vi "FipsAdjacent.vi"() -> (11 "Fips":i32[](array[numeric]))   [LabVIEW 2017] (continued)
TN\"\t47041\n\"Warren County, TN\"\t47177\t\"Grundy County, TN\"\t47061\n\"Warren County, TN\"\t47177\t\"Sequatchie County, TN\"\t47153\n\"Warren County, TN\"\t47177\t\"Van Buren County, TN\"\t47175\n\"Warren County, TN\"\t47177\t\"Warren County, TN\"\t47177\n\"Warren County, TN\"\t47177\t\"White County, TN\"\t47185\n\"Washington County, TN\"\t47179\t\"Carter County, TN\"\t47019\n\"Washington County, TN\"\t47179\t\"Greene County, TN\"\t47059\n\"Washington County, TN\"\t47179\t\"Hawkins County, TN\"\t47073\n\"Washington County, TN\"\t47179\t\"Sullivan County, TN\"\t47163\n\"Washington County, TN\"\t47179\t\"Unicoi County, TN\"\t47171\n\"Washington County, TN\"\t47179\t\"Washington County, TN\"\t47179\n\"Wayne County, TN\"\t47181\t\"Lauderdale County, AL\"\t01077\n\"Wayne County, TN\"\t47181\t\"Decatur County, TN\"\t47039\n\"Wayne County, TN\"\t47181\t\"Hardin County, TN\"\t47071\n\"Wayne County, TN\"\t47181\t\"Lawrence County, TN\"\t47099\n\"Wayne County, TN\"\t47181\t\"Lewis County, TN\"\t47101\n\"Wayne County, TN\"\t47181\t\"Perry County, TN\"\t47135\n\"Wayne County, TN\"\t47181\t\"Wayne County, TN\"\t47181\n\"Weakley County, TN\"\t47183\t\"Graves County, KY\"\t21083\n\"Weakley County, TN\"\t47183\t\"Hickman County, KY\"\t21105\n\"Weakley County, TN\"\t47183\t\"Carroll County, TN\"\t47017\n\"Weakley County, TN\"\t47183\t\"Gibson County, TN\"\t47053\n\"Weakley County, TN\"\t47183\t\"Henry County, TN\"\t47079\n\"Weakley County, TN\"\t47183\t\"Obion County, TN\"\t47131\n\"Weakley County, TN\"\t47183\t\"Weakley County, TN\"\t47183\n\"White County, TN\"\t47185\t\"Cumberland County, TN\"\t47035\n\"White County, TN\"\t47185\t\"DeKalb County, TN\"\t47041\n\"White County, TN\"\t47185\t\"Putnam County, TN\"\t47141\n\"White County, TN\"\t47185\t\"Van Buren County, TN\"\t47175\n\"White County, TN\"\t47185\t\"Warren County, TN\"\t47177\n\"White County, TN\"\t47185\t\"White County, TN\"\t47185\n\"Williamson County, TN\"\t47187\t\"Cheatham County, TN\"\t47021\n\"Williamson County, TN\"\t47187\t\"Davidson County, TN\"\t47037\n\"Williamson County, TN\"\t47187\t\"Dickson County, TN\"\t47043\n\"Williamson County, TN\"\t47187\t\"Hickman County, TN\"\t47081\n\"Williamson County, TN\"\t47187\t\"Marshall County, TN\"\t47117\n\"Williamson County, TN\"\t47187\t\"Maury County, TN\"\t47119\n\"Williamson County, TN\"\t47187\t\"Rutherford County, TN\"\t47149\n\"Williamson County, TN\"\t47187\t\"Williamson County, TN\"\t47187\n\"Wilson County, TN\"\t47189\t\"Cannon County, TN\"\t47015\n\"Wilson County, TN\"\t47189\t\"Davidson County, TN\"\t47037\n\"Wilson County, TN\"\t47189\t\"DeKalb County, TN\"\t47041\n\"Wilson County, TN\"\t47189\t\"Rutherford County, TN\"\t47149\n\"Wilson County, TN\"\t47189\t\"Smith County, TN\"\t47159\n\"Wilson County, TN\"\t47189\t\"Sumner County, TN\"\t47165\n\"Wilson County, TN\"\t47189\t\"Trousdale County, TN\"\t47169\n\"Wilson County, TN\"\t47189\t\"Wilson County, TN\"\t47189\n\"Anderson County, TX\"\t48001\t\"Anderson County, TX\"\t48001\n\"Anderson County, TX\"\t48001\t\"Cherokee County, TX\"\t48073\n\"Anderson County, TX\"\t48001\t\"Freestone County, TX\"\t48161\n\"Anderson County, TX\"\t48001\t\"Henderson County, TX\"\t48213\n\"Anderson County, TX\"\t48001\t\"Houston County, TX\"\t48225\n\"Anderson County, TX\"\t48001\t\"Leon County, TX\"\t48289\n\"Andrews County, TX\"\t48003\t\"Lea County, NM\"\t35025\n\"Andrews County, TX\"\t48003\t\"Andrews County, TX\"\t48003\n\"Andrews County, TX\"\t48003\t\"Ector County, TX\"\t48135\n\"Andrews County, TX\"\t48003\t\"Gaines County, TX\"\t48165\n\"Andrews County, TX\"\t48003\t\"Martin County, TX\"\t48317\n\"Andrews County, TX\"\t48003\t\"Midland County, TX\"\t48329\n\"Andrews County, TX\"\t48003\t\"Winkler County, TX\"\t48495\n\"Angelina County, TX\"\t48005\t\"Angelina County, TX\"\t48005\n\"Angelina County, TX\"\t48005\t\"Cherokee County, TX\"\t48073\n\"Angelina County, TX\"\t48005\t\"Houston County, TX\"\t48225\n\"Angelina County, TX\"\t48005\t\"Jasper County, TX\"\t48241\n\"Angelina County, TX\"\t48005\t\"Nacogdoches County, TX\"\t48347\n\"Angelina County, TX\"\t48005\t\"Polk County, TX\"\t48373\n\"Angelina County, TX\"\t48005\t\"San Augustine County, TX\"\t48405\n\"Angelina County, TX\"\t48005\t\"Trinity County, TX\"\t48455\n\"Angelina County, TX\"\t48005\t\"Tyler County, TX\"\t48457\n\"Aransas County, TX\"\t48007\t\"Aransas County, TX\"\t48007\n\"Aransas County, TX\"\t48007\t\"Calhoun County, TX\"\t48057\n\"Aransas County, TX\"\t48007\t\"Nueces County, TX\"\t48355\n\"Aransas County, TX\"\t48007\t\"Refugio County, TX\"\t48391\n\"Aransas County, TX\"\t48007\t\"San Patricio County, TX\"\t48409\n\"Archer County, TX\"\t48009\t\"Archer County, TX\"\t48009\n\"Archer County, TX\"\t48009\t\"Baylor County, TX\"\t48023\n\"Archer County, TX\"\t48009\t\"Clay County, TX\"\t48077\n\"Archer County, TX\"\t48009\t\"Jack County, TX\"\t48237\n\"Archer County, TX\"\t48009\t\"Throckmorton County, TX\"\t48447\n\"Archer County, TX\"\t48009\t\"Wichita County, TX\"\t48485\n\"Archer County, TX\"\t48009\t\"Wilbarger County, TX\"\t48487\n\"Archer County, TX\"\t48009\t\"Young County, TX\"\t48503\n\"Armstrong County, TX\"\t48011\t\"Armstrong County, TX\"\t48011\n\"Armstrong County, TX\"\t48011\t\"Briscoe County, TX\"\t48045\n\"Armstrong County, TX\"\t48011\t\"Carson County, TX\"\t48065\n\"Armstrong County, TX\"\t48011\t\"Donley County, TX\"\t48129\n\"Armstrong County, TX\"\t48011\t\"Gray County, TX\"\t48179\n\"Armstrong County, TX\"\t48011\t\"Potter County, TX\"\t48375\n\"Armstrong County, TX\"\t48011\t\"Randall County, TX\"\t48381\n\"Armstrong County, TX\"\t48011\t\"Swisher County, TX\"\t48437\n\"Atascosa County, TX\"\t48013\t\"Atascosa County, TX\"\t48013\n\"Atascosa County, TX\"\t48013\t\"Bexar County, TX\"\t48029\n\"Atascosa County, TX\"\t48013\t\"Frio County, TX\"\t48163\n\"Atascosa County, TX\"\t48013\t\"Karnes County, TX\"\t48255\n\"Atascosa County, TX\"\t48013\t\"La Salle County, TX\"\t48283\n\"Atascosa County, TX\"\t48013\t\"Live Oak County, TX\"\t48297\n\"Atascosa County, TX\"\t48013\t\"McMullen County, TX\"\t48311\n\"Atascosa County, TX\"\t48013\t\"Medina County, TX\"\t48325\n\"Atascosa County, TX\"\t48013\t\"Wilson County, TX\"\t48493\n\"Austin County, TX\"\t48015\t\"Austin County, TX\"\t48015\n\"Austin County, TX\"\t48015\t\"Colorado County, TX\"\t48089\n\"Austin County, TX\"\t48015\t\"Fayette County, TX\"\t48149\n\"Austin County, TX\"\t48015\t\"Fort Bend County, TX\"\t48157\n\"Austin County, TX\"\t48015\t\"Waller County, TX\"\t48473\n\"Austin County, TX\"\t48015\t\"Washington County, TX\"\t48477\n\"Austin County, TX\"\t48015\t\"Wharton County, TX\"\t48481\n\"Bailey County, TX\"\t48017\t\"Curry County, NM\"\t35009\n\"Bailey County, TX\"\t48017\t\"Roosevelt County, NM\"\t35041\n\"Bailey County, TX\"\t48017\t\"Bailey County, TX\"\t48017\n\"Bailey County, TX\"\t48017\t\"Cochran County, TX\"\t48079\n\"Bailey County, TX\"\t48017\t\"Hockley County, TX\"\t48219\n\"Bailey County, TX\"\t48017\t\"Lamb County, TX\"\t48279\n\"Bailey County, TX\"\t48017\t\"Parmer County, TX\"\t48369\n\"Bandera County, TX\"\t48019\t\"Bandera County, TX\"\t48019\n\"Bandera County, TX\"\t48019\t\"Bexar County, TX\"\t48029\n\"Bandera County, TX\"\t48019\t\"Kendall County, TX\"\t48259\n\"Bandera County, TX\"\t48019\t\"Kerr County, TX\"\t48265\n\"Bandera County, TX\"\t48019\t\"Medina County, TX\"\t48325\n\"Bandera County, TX\"\t48019\t\"Real County, TX\"\t48385\n\"Bandera County, TX\"\t48019\t\"Uvalde County, TX\"\t48463\n\"Bastrop County, TX\"\t48021\t\"Bastrop County, TX\"\t48021\n\"Bastrop County, TX\"\t48021\t\"Caldwell County, TX\"\t48055\n\"Bastrop County, TX\"\t48021\t\"Fayette County, TX\"\t48149\n\"Bastrop County, TX\"\t48021\t\"Lee County, TX\"\t48287\n\"Bastrop County, TX\"\t48021\t\"Travis County, TX\"\t48453\n\"Bastrop County, TX\"\t48021\t\"Williamson County, TX\"\t48491\n\"Baylor County, TX\"\t48023\t\"Archer County, TX\"\t48009\n\"Baylor County, TX\"\t48023\t\"Baylor County, TX\"\t48023\n\"Baylor County, TX\"\t48023\t\"Foard County, TX\"\t48155\n\"Baylor County, TX\"\t48023\t\"Haskell County, TX\"\t48207\n\"Baylor County, TX\"\t48023\t\"Knox County, TX\"\t48275\n\"Baylor County, TX\"\t48023\t\"Throckmorton County, TX\"\t48447\n\"Baylor County, TX\"\t48023\t\"Wichita County, TX\"\t48485\n\"Baylor County, TX\"\t48023\t\"Wilbarger County, TX\"\t48487\n\"Baylor County, TX\"\t48023\t\"Young County, TX\"\t48503\n\"Bee County, TX\"\t48025\t\"Bee County, TX\"\t48025\n\"Bee County, TX\"\t48025\t\"Goliad County, TX\"\t48175\n\"Bee County, TX\"\t48025\t\"Karnes County, TX\"\t48255\n\"Bee County, TX\"\t48025\t\"Live Oak County, TX\"\t48297\n\"Bee County, TX\"\t48025\t\"Refugio County, TX\"\t48391\n\"Bee County, TX\"\t48025\t\"San Patricio County, TX\"\t48409\n\"Bell County, TX\"\t48027\t\"Bell County, TX\"\t48027\n\"Bell County, TX\"\t48027\t\"Burnet County, TX\"\t48053\n\"Bell County, TX\"\t48027\t\"Coryell County, TX\"\t48099\n\"Bell County, TX\"\t48027\t\"Falls County, TX\"\t48145\n\"Bell County, TX\"\t48027\t\"Lampasas County, TX\"\t48281\n\"Bell County, TX\"\t48027\t\"McLennan County, TX\"\t48309\n\"Bell County, TX\"\t48027\t\"Milam County, TX\"\t48331\n\"Bell County, TX\"\t48027\t\"Williamson County, TX\"\t48491\n\"Bexar County, TX\"\t48029\t\"Atascosa County, TX\"\t48013\n\"Bexar County, TX\"\t48029\t\"Bandera County, TX\"\t48019\n\"Bexar County, TX\"\t48029\t\"Bexar County, TX\"\t48029\n\"Bexar County, TX\"\t48029\t\"Comal County, TX\"\t48091\n\"Bexar County, TX\"\t48029\t\"Guadalupe County, TX\"\t48187\n\"Bexar County, TX\"\t48029\t\"Kendall County, TX\"\t48259\n\"Bexar County, TX\"\t48029\t\"Medina County, TX\"\t48325\n\"Bexar County, TX\"\t48029\t\"Wilson County, TX\"\t48493\n\"Blanco County, TX\"\t48031\t\"Blanco County, TX\"\t48031\n\"Blanco County, TX\"\t48031\t\"Burnet County, TX\"\t48053\n\"Blanco County, TX\"\t48031\t\"Comal County, TX\"\t48091\n\"Blanco County, TX\"\t48031\t\"Gillespie County, TX\"\t48171\n\"Blanco County, TX\"\t48031\t\"Hays County, TX\"\t48209\n\"Blanco County, TX\"\t48031\t\"Kendall County, TX\"\t48259\n\"Blanco County, TX\"\t48031\t\"Llano County, TX\"\t48299\n\"Blanco County, TX\"\t48031\t\"Travis County, TX\"\t48453\n\"Borden County, TX\"\t48033\t\"Borden County, TX\"\t48033\n\"Borden County, TX\"\t48033\t\"Dawson County, TX\"\t48115\n\"Borden County, TX\"\t48033\t\"Garza County, TX\"\t48169\n\"Borden County, TX\"\t48033\t\"Howard County, TX\"\t48227\n\"Borden County, TX\"\t48033\t\"Lynn County, TX\"\t48305\n\"Borden County, TX\"\t48033\t\"Martin County, TX\"\t48317\n\"Borden County, TX\"\t48033\t\"Mitchell County, TX\"\t48335\n\"Borden County, TX\"\t48033\t\"Scurry County, TX\"\t48415\n\"Bosque County, TX\"\t48035\t\"Bosque County, TX\"\t48035\n\"Bosque County, TX\"\t48035\t\"Coryell County, TX\"\t48099\n\"Bosque County, TX\"\t48035\t\"Erath County, TX\"\t48143\n\"Bosque County, TX\"\t48035\t\"Hamilton County, TX\"\t48193\n\"Bosque County, TX\"\t48035\t\"Hill County, TX\"\t48217\n\"Bosque County, TX\"\t48035\t\"Johnson County, TX\"\t48251\n\"Bosque County, TX\"\t48035\t\"McLennan County, TX\"\t48309\n\"Bosque County, TX\"\t48035\t\"Somervell County, TX\"\t48425\n\"Bowie County, TX\"\t48037\t\"Little River County, AR\"\t05081\n\"Bowie County, TX\"\t48037\t\"Miller County, AR\"\t05091\n\"Bowie County, TX\"\t48037\t\"McCurtain County, OK\"\t40089\n\"Bowie County, TX\"\t48037\t\"Bowie County, TX\"\t48037\n\"Bowie County, TX\"\t48037\t\"Cass County, TX\"\t48067\n\"Bowie County, TX\"\t48037\t\"Morris County, TX\"\t48343\n\"Bowie County, TX\"\t48037\t\"Red River County, TX\"\t48387\n\"Brazoria County, TX\"\t48039\t\"Brazoria County, TX\"\t48039\n\"Brazoria County, TX\"\t48039\t\"Fort Bend County, TX\"\t48157\n\"Brazoria County, TX\"\t48039\t\"Galveston County, TX\"\t48167\n\"Brazoria County, TX\"\t48039\t\"Harris County, TX\"\t48201\n\"Brazoria County, TX\"\t48039\t\"Matagorda County, TX\"\t48321\n\"Brazoria County, TX\"\t48039\t\"Wharton County, TX\"\t48481\n\"Brazos County, TX\"\t48041\t\"Brazos County, TX\"\t48041\n\"Brazos County, TX\"\t48041\t\"Burleson County, TX\"\t48051\n\"Brazos County, TX\"\t48041\t\"Grimes County, TX\"\t48185\n\"Brazos County, TX\"\t48041\t\"Leon County, TX\"\t48289\n\"Brazos County, TX\"\t48041\t\"Madison County, TX\"\t48313\n\"Brazos County, TX\"\t48041\t\"Robertson County, TX\"\t48395\n\"Brazos County, TX\"\t48041\t\"Washington County, TX\"\t48477\n\"Brewster County, TX\"\t48043\t\"Brewster County, TX\"\t48043\n\"Brewster County, TX\"\t48043\t\"Jeff Davis County, TX\"\t48243\n\"Brewster County, TX\"\t48043\t\"Pecos County, TX\"\t48371\n\"Brewster County, TX\"\t48043\t\"Presidio County, TX\"\t48377\n\"Brewster County, TX\"\t48043\t\"Terrell County, TX\"\t48443\n\"Briscoe County, TX\"\t48045\t\"Armstrong County, TX\"\t48011\n\"Briscoe County, TX\"\t48045\t\"Briscoe County, TX\"\t48045\n\"Briscoe County, TX\"\t48045\t\"Donley County, TX\"\t48129\n\"Briscoe County, TX\"\t48045\t\"Floyd County, TX\"\t48153\n\"Briscoe County, TX\"\t48045\t\"Hall County, TX\"\t48191\n\"Briscoe County, TX\"\t48045\t\"Motley County, TX\"\t48345\n\"Briscoe County, TX\"\t48045\t\"Swisher County, TX\"\t48437\n\"Brooks County, TX\"\t48047\t\"Brooks County, TX\"\t48047\n\"Brooks County, TX\"\t48047\t\"Duval County, TX\"\t48131\n\"Brooks County, TX\"\t48047\t\"Hidalgo County, TX\"\t48215\n\"Brooks County, TX\"\t48047\t\"Jim Hogg County, TX\"\t48247\n\"Brooks County, TX\"\t48047\t\"Jim Wells County, TX\"\t48249\n\"Brooks County, TX\"\t48047\t\"Kenedy County, TX\"\t48261\n\"Brooks County, TX\"\t48047\t\"Kleberg County, TX\"\t48273\n\"Brooks County, TX\"\t48047\t\"Starr County, TX\"\t48427\n\"Brown County, TX\"\t48049\t\"Brown County, TX\"\t48049\n\"Brown County, TX\"\t48049\t\"Callahan County, TX\"\t48059\n\"Brown County, TX\"\t48049\t\"Coleman County, TX\"\t48083\n\"Brown County, TX\"\t48049\t\"Comanche County, TX\"\t48093\n\"Brown County, TX\"\t48049\t\"Eastland County, TX\"\t48133\n\"Brown County, TX\"\t48049\t\"McCulloch County, TX\"\t48307\n\"Brown County, TX\"\t48049\t\"Mills County, TX\"\t48333\n\"Brown County, TX\"\t48049\t\"San Saba County, TX\"\t48411\n\"Burleson County, TX\"\t48051\t\"Brazos County, TX\"\t48041\n\"Burleson County, TX\"\t48051\t\"Burleson County, TX\"\t48051\n\"Burleson County, TX\"\t48051\t\"Lee County, TX\"\t48287\n\"Burleson County, TX\"\t48051\t\"Milam County, TX\"\t48331\n\"Burleson County, TX\"\t48051\t\"Robertson County, TX\"\t48395\n\"Burleson County, TX\"\t48051\t\"Washington County, TX\"\t48477\n\"Burnet County, TX\"\t48053\t\"Bell County, TX\"\t48027\n\"Burnet County, TX\"\t48053\t\"Blanco County, TX\"\t48031\n\"Burnet County, TX\"\t48053\t\"Burnet County, TX\"\t48053\n\"Burnet County, TX\"\t48053\t\"Lampasas County, TX\"\t48281\n\"Burnet County, TX\"\t48053\t\"Llano County, TX\"\t48299\n\"Burnet County, TX\"\t48053\t\"San Saba County, TX\"\t48411\n\"Burnet County, TX\"\t48053\t\"Travis County, TX\"\t48453\n\"Burnet County, TX\"\t48053\t\"Williamson County, TX\"\t48491\n\"Caldwell County, TX\"\t48055\t\"Bastrop County, TX\"\t48021\n\"Caldwell County, TX\"\t48055\t\"Caldwell County, TX\"\t48055\n\"Caldwell County, TX\"\t48055\t\"Fayette County, TX\"\t48149\n\"Caldwell County, TX\"\t48055\t\"Gonzales County, TX\"\t48177\n\"Caldwell County, TX\"\t48055\t\"Guadalupe County, TX\"\t48187\n\"Caldwell County, TX\"\t48055\t\"Hays County, TX\"\t48209\n\"Caldwell County, TX\"\t48055\t\"Travis County, TX\"\t48453\n\"Calhoun County, TX\"\t48057\t\"Aransas County, TX\"\t48007\n\"Calhoun County, TX\"\t48057\t\"Calhoun County, TX\"\t48057\n\"Calhoun County, TX\"\t48057\t\"Jackson County, TX\"\t48239\n\"Calhoun County, TX\"\t48057\t\"Matagorda County, TX\"\t48321\n\"Calhoun County, TX\"\t48057\t\"Refugio County, TX\"\t48391\n\"Calhoun County, TX\"\t48057\t\"Victoria County, TX\"\t48469\n\"Callahan County, TX\"\t48059\t\"Brown County, TX\"\t48049\n\"Callahan County, TX\"\t48059\t\"Callahan County, TX\"\t48059\n\"Callahan County, TX\"\t48059\t\"Coleman County, TX\"\t48083\n\"Callahan County, TX\"\t48059\t\"Eastland County, TX\"\t48133\n\"Callahan County, TX\"\t48059\t\"Jones County, TX\"\t48253\n\"Callahan County, TX\"\t48059\t\"Shackelford County, TX\"\t48417\n\"Callahan County, TX\"\t48059\t\"Taylor County, TX\"\t48441\n\"Cameron County, TX\"\t48061\t\"Cameron County, TX\"\t48061\n\"Cameron County, TX\"\t48061\t\"Hidalgo County, TX\"\t48215\n\"Cameron County, TX\"\t48061\t\"Willacy County, TX\"\t48489\n\"Camp County, TX\"\t48063\t\"Camp County, TX\"\t48063\n\"Camp County, TX\"\t48063\t\"Franklin County, TX\"\t48159\n\"Camp County, TX\"\t48063\t\"Morris County, TX\"\t48343\n\"Camp County, TX\"\t48063\t\"Titus County, TX\"\t48449\n\"Camp County, TX\"\t48063\t\"Upshur County, TX\"\t48459\n\"Camp County, TX\"\t48063\t\"Wood County, TX\"\t48499\n\"Carson County, TX\"\t48065\t\"Armstrong County, TX\"\t48011\n\"Carson County, TX\"\t48065\t\"Carson County, TX\"\t48065\n\"Carson County, TX\"\t48065\t\"Donley County, TX\"\t48129\n\"Carson County, TX\"\t48065\t\"Gray County, TX\"\t48179\n\"Carson County, TX\"\t48065\t\"Hutchinson County, TX\"\t48233\n\"Carson County, TX\"\t48065\t\"Moore County, TX\"\t48341\n\"Carson County, TX\"\t48065\t\"Potter County, TX\"\t48375\n\"Carson County, TX\"\t48065\t\"Randall County, TX\"\t48381\n\"Carson County, TX\"\t48065\t\"Roberts County, TX\"\t48393\n\"Cass County, TX\"\t48067\t\"Miller County, AR\"\t05091\n\"Cass County, TX\"\t48067\t\"Caddo Parish, LA\"\t22017\n\"Cass County, TX\"\t48067\t\"Bowie County, TX\"\t48037\n\"Cass County, TX\"\t48067\t\"Cass County, TX\"\t48067\n\"Cass County, TX\"\t48067\t\"Marion County, TX\"\t48315\n\"Cass County, TX\"\t48067\t\"Morris County, TX\"\t48343\n\"Castro County, TX\"\t48069\t\"Castro County, TX\"\t48069\n\"Castro County, TX\"\t48069\t\"Deaf Smith County, TX\"\t48117\n\"Castro County, TX\"\t48069\t\"Hale County, TX\"\t48189\n\"Castro County, TX\"\t48069\t\"Lamb County, TX\"\t48279\n\"Castro County, TX\"\t48069\t\"Parmer County, TX\"\t48369\n\"Castro County, TX\"\t48069\t\"Randall County, TX\"\t48381\n\"Castro County, TX\"\t48069\t\"Swisher County, TX\"\t48437\n\"Chambers County, TX\"\t48071\t\"Chambers County, TX\"\t48071\n\"Chambers County, TX\"\t48071\t\"Galveston County, TX\"\t48167\n\"Chambers County, TX\"\t48071\t\"Harris County, TX\"\t48201\n\"Chambers County, TX\"\t48071\t\"Jefferson County, TX\"\t48245\n\"Chambers County, TX\"\t48071\t\"Liberty County, TX\"\t48291\n\"Cherokee County, TX\"\t48073\t\"Anderson County, TX\"\t48001\n\"Cherokee County, TX\"\t48073\t\"Angelina County, TX\"\t48005\n\"Cherokee County, TX\"\t48073\t\"Cherokee County, TX\"\t48073\n\"Cherokee County, TX\"\t48073\t\"Henderson County, TX\"\t48213\n\"Cherokee County, TX\"\t48073\t\"Houston County, TX\"\t48225\n\"Cherokee County, TX\"\t48073\t\"Nacogdoches County, TX\"\t48347\n\"Cherokee County, TX\"\t48073\t\"Rusk County, TX\"\t48401\n\"Cherokee County, TX\"\t48073\t\"Smith County, TX\"\t48423\n\"Childress County, TX\"\t48075\t\"Harmon County, OK\"\t40057\n\"Childress County, TX\"\t48075\t\"Childress County, TX\"\t48075\n\"Childress County, TX\"\t48075\t\"Collingsworth County, TX\"\t48087\n\"Childress County, TX\"\t48075\t\"Cottle County, TX\"\t48101\n\"Childress County, TX\"\t48075\t\"Hall County, TX\"\t48191\n\"Childress County, TX\"\t48075\t\"Hardeman County, TX\"\t48197\n\"Clay County, TX\"\t48077\t\"Cotton County, OK\"\t40033\n\"Clay County, TX\"\t48077\t\"Jefferson County, OK\"\t40067\n\"Clay County, TX\"\t48077\t\"Archer County, TX\"\t48009\n\"Clay County, TX\"\t48077\t\"Clay County, TX\"\t48077\n\"Clay County, TX\"\t48077\t\"Jack County, TX\"\t48237\n\"Clay County, TX\"\t48077\t\"Montague County, TX\"\t48337\n\"Clay County, TX\"\t48077\t\"Wichita County, TX\"\t48485\n\"Cochran County, TX\"\t48079\t\"Lea County, NM\"\t35025\n\"Cochran County, TX\"\t48079\t\"Roosevelt County, NM\"\t35041\n\"Cochran County, TX\"\t48079\t\"Bailey County, TX\"\t48017\n\"Cochran County, TX\"\t48079\t\"Cochran County, TX\"\t48079\n\"Cochran County, TX\"\t48079\t\"Hockley County, TX\"\t48219\n\"Cochran County, TX\"\t48079\t\"Lamb County, TX\"\t48279\n\"Cochran County, TX\"\t48079\t\"Terry County, TX\"\t48445\n\"Cochran County, TX\"\t48079\t\"Yoakum County, TX\"\t48501\n\"Coke County, TX\"\t48081\t\"Coke County, TX\"\t48081\n\"Coke County, TX\"\t48081\t\"Mitchell County, TX\"\t48335\n\"Coke County, TX\"\t48081\t\"Nolan County, TX\"\t48353\n\"Coke County, TX\"\t48081\t\"Runnels County, TX\"\t48399\n\"Coke County, TX\"\t48081\t\"Sterling County, TX\"\t48431\n\"Coke County, TX\"\t48081\t\"Tom Green County, TX\"\t48451\n\"Coleman County, TX\"\t48083\t\"Brown County, TX\"\t48049\n\"Coleman County, TX\"\t48083\t\"Callahan County, TX\"\t48059\n\"Coleman County, TX\"\t48083\t\"Coleman County, TX\"\t48083\n\"Coleman County, TX\"\t48083\t\"Concho County, TX\"\t48095\n\"Coleman County, TX\"\t48083\t\"McCulloch County, TX\"\t48307\n\"Coleman County, TX\"\t48083\t\"Runnels County, TX\"\t48399\n\"Coleman County, TX\"\t48083\t\"Taylor County, TX\"\t48441\n\"Collin County, TX\"\t48085\t\"Collin County, TX\"\t48085\n\"Collin County, TX\"\t48085\t\"Dallas County, TX\"\t48113\n\"Collin County, TX\"\t48085\t\"Denton County, TX\"\t48121\n\"Collin County, TX\"\t48085\t\"Fannin County, TX\"\t48147\n\"Collin County, TX\"\t48085\t\"Grayson County, TX\"\t48181\n\"Collin County, TX\"\t48085\t\"Hunt County, TX\"\t48231\n\"Collin County, TX\"\t48085\t\"Rockwall County, TX\"\t48397\n\"Collingsworth County, TX\"\t48087\t\"Beckham County, OK\"\t40009\n\"Collingsworth County, TX\"\t48087\t\"Harmon County, OK\"\t40057\n\"Collingsworth County, TX\"\t48087\t\"Childress County, TX\"\t48075\n\"Collingsworth County, TX\"\t48087\t\"Collingsworth County, TX\"\t48087\n\"Collingsworth County, TX\"\t48087\t\"Donley County, TX\"\t48129\n\"Collingsworth County, TX\"\t48087\t\"Gray County, TX\"\t48179\n\"Collingsworth County, TX\"\t48087\t\"Hall County, TX\"\t48191\n\"Collingsworth County, TX\"\t48087\t\"Wheeler County, TX\"\t48483\n\"Colorado County, TX\"\t48089\t\"Austin County, TX\"\t48015\n\"Colorado County, TX\"\t48089\t\"Colorado County, TX\"\t48089\n\"Colorado County, TX\"\t48089\t\"Fayette County, TX\"\t48149\n\"Colorado County, TX\"\t48089\t\"Jackson County, TX\"\t48239\n\"Colorado County, TX\"\t48089\t\"Lavaca County, TX\"\t48285\n\"Colorado County, TX\"\t48089\t\"Wharton County, TX\"\t48481\n\"Comal County, TX\"\t48091\t\"Bexar County, TX\"\t48029\n\"Comal County, TX\"\t48091\t\"Blanco County, TX\"\t48031\n\"Comal County, TX\"\t48091\t\"Comal County, TX\"\t48091\n\"Comal County, TX\"\t48091\t\"Guadalupe County, TX\"\t48187\n\"Comal County, TX\"\t48091\t\"Hays County, TX\"\t48209\n\"Comal County, TX\"\t48091\t\"Kendall County, TX\"\t48259\n\"Comanche County, TX\"\t48093\t\"Brown County, TX\"\t48049\n\"Comanche County, TX\"\t48093\t\"Comanche County, TX\"\t48093\n\"Comanche County, TX\"\t48093\t\"Eastland County, TX\"\t48133\n\"Comanche County, TX\"\t48093\t\"Erath County, TX\"\t48143\n\"Comanche County, TX\"\t48093\t\"Hamilton County, TX\"\t48193\n\"Comanche County, TX\"\t48093\t\"Mills County, TX\"\t48333\n\"Concho County, TX\"\t48095\t\"Coleman County, TX\"\t48083\n\"Concho County, TX\"\t48095\t\"Concho County, TX\"\t48095\n\"Concho County, TX\"\t48095\t\"McCulloch County, TX\"\t48307\n\"Concho County, TX\"\t48095\t\"Menard County, TX\"\t48327\n\"Concho County, TX\"\t48095\t\"Runnels County, TX\"\t48399\n\"Concho County, TX\"\t48095\t\"Schleicher County, TX\"\t48413\n\"Concho County, TX\"\t48095\t\"Tom Green County, TX\"\t48451\n\"Cooke County, TX\"\t48097\t\"Love County, OK\"\t40085\n\"Cooke County, TX\"\t48097\t\"Cooke County, TX\"\t48097\n\"Cooke County, TX\"\t48097\t\"Denton County, TX\"\t48121\n\"Cooke County, TX\"\t48097\t\"Grayson County, TX\"\t48181\n\"Cooke County, TX\"\t48097\t\"Montague County, TX\"\t48337\n\"Cooke County, TX\"\t48097\t\"Wise County, TX\"\t48497\n\"Coryell County, TX\"\t48099\t\"Bell County, TX\"\t48027\n\"Coryell County, TX\"\t48099\t\"Bosque County, TX\"\t48035\n\"Coryell County, TX\"\t48099\t\"Coryell County, TX\"\t48099\n\"Coryell County, TX\"\t48099\t\"Hamilton County, TX\"\t48193\n\"Coryell County, TX\"\t48099\t\"Lampasas County, TX\"\t48281\n\"Coryell County, TX\"\t48099\t\"McLennan County, TX\"\t48309\n\"Cottle County, TX\"\t48101\t\"Childress County, TX\"\t48075\n\"Cottle County, TX\"\t48101\t\"Cottle County, TX\"\t48101\n\"Cottle County, TX\"\t48101\t\"Dickens County, TX\"\t48125\n\"Cottle County, TX\"\t48101\t\"Foard County, TX\"\t48155\n\"Cottle County, TX\"\t48101\t\"Hall County, TX\"\t48191\n\"Cottle County, TX\"\t48101\t\"Hardeman County, TX\"\t48197\n\"Cottle County, TX\"\t48101\t\"King County, TX\"\t48269\n\"Cottle County, TX\"\t48101\t\"Motley County, TX\"\t48345\n\"Crane County, TX\"\t48103\t\"Crane County, TX\"\t48103\n\"Crane County, TX\"\t48103\t\"Crockett County, TX\"\t48105\n\"Crane County, TX\"\t48103\t\"Ector County, TX\"\t48135\n\"Crane County, TX\"\t48103\t\"Pecos County, TX\"\t48371\n\"Crane County, TX\"\t48103\t\"Upton County, TX\"\t48461\n\"Crane County, TX\"\t48103\t\"Ward County, TX\"\t48475\n\"Crockett County, TX\"\t48105\t\"Crane County, TX\"\t48103\n\"Crockett County, TX\"\t48105\t\"Crockett County, TX\"\t48105\n\"Crockett County, TX\"\t48105\t\"Irion County, TX\"\t48235\n\"Crockett County, TX\"\t48105\t\"Pecos County, TX\"\t48371\n\"Crockett County, TX\"\t48105\t\"Reagan County, TX\"\t48383\n\"Crockett County, TX\"\t48105\t\"Schleicher County, TX\"\t48413\n\"Crockett County, TX\"\t48105\t\"Sutton County, TX\"\t48435\n\"Crockett County, TX\"\t48105\t\"Terrell County, TX\"\t48443\n\"Crockett County, TX\"\t48105\t\"Upton County, TX\"\t48461\n\"Crockett County, TX\"\t48105\t\"Val Verde County, TX\"\t48465\n\"Crosby County, TX\"\t48107\t\"Crosby County, TX\"\t48107\n\"Crosby County, TX\"\t48107\t\"Dickens County, TX\"\t48125\n\"Crosby County, TX\"\t48107\t\"Floyd County, TX\"\t48153\n\"Crosby County, TX\"\t48107\t\"Garza County, TX\"\t48169\n\"Crosby County, TX\"\t48107\t\"Hale County, TX\"\t48189\n\"Crosby County, TX\"\t48107\t\"Kent County, TX\"\t48263\n\"Crosby County, TX\"\t48107\t\"Lubbock County, TX\"\t48303\n\"Crosby County, TX\"\t48107\t\"Lynn County, TX\"\t48305\n\"Crosby County, TX\"\t48107\t\"Motley County, TX\"\t48345\n\"Culberson County, TX\"\t48109\t\"Eddy County, NM\"\t35015\n\"Culberson County, TX\"\t48109\t\"Otero County, NM\"\t35035\n\"Culberson County, TX\"\t48109\t\"Culberson County, TX\"\t48109\n\"Culberson County, TX\"\t48109\t\"Hudspeth County, TX\"\t48229\n\"Culberson County, TX\"\t48109\t\"Jeff Davis County, TX\"\t48243\n\"Culberson County, TX\"\t48109\t\"Reeves County, TX\"\t48389\n\"Dallam County, TX\"\t48111\t\"Union County, NM\"\t35059\n\"Dallam County, TX\"\t48111\t\"Cimarron County, OK\"\t40025\n\"Dallam County, TX\"\t48111\t\"Dallam County, TX\"\t48111\n\"Dallam County, TX\"\t48111\t\"Hartley County, TX\"\t48205\n\"Dallam County, TX\"\t48111\t\"Moore County, TX\"\t48341\n\"Dallam County, TX\"\t48111\t\"Sherman County, TX\"\t48421\n\"Dallas County, TX\"\t48113\t\"Collin County, TX\"\t48085\n\"Dallas County, TX\"\t48113\t\"Dallas County, TX\"\t48113\n\"Dallas County, TX\"\t48113\t\"Denton County, TX\"\t48121\n\"Dallas County, TX\"\t48113\t\"Ellis County, TX\"\t48139\n\"Dallas County, TX\"\t48113\t\"Kaufman County, TX\"\t48257\n\"Dallas County, TX\"\t48113\t\"Rockwall County, TX\"\t48397\n\"Dallas County, TX\"\t48113\t\"Tarrant County, TX\"\t48439\n\"Dawson County, TX\"\t48115\t\"Borden County, TX\"\t48033\n\"Dawson County, TX\"\t48115\t\"Dawson County, TX\"\t48115\n\"Dawson County, TX\"\t48115\t\"Gaines County, TX\"\t48165\n\"Dawson County, TX\"\t48115\t\"Howard County, TX\"\t48227\n\"Dawson County, TX\"\t48115\t\"Lynn County, TX\"\t48305\n\"Dawson County, TX\"\t48115\t\"Martin County, TX\"\t48317\n\"Dawson County, TX\"\t48115\t\"Terry County, TX\"\t48445\n\"Deaf Smith County, TX\"\t48117\t\"Curry County, NM\"\t35009\n\"Deaf Smith County, TX\"\t48117\t\"Quay County, NM\"\t35037\n\"Deaf Smith County, TX\"\t48117\t\"Castro County, TX\"\t48069\n\"Deaf Smith County, TX\"\t48117\t\"Deaf Smith County, TX\"\t48117\n\"Deaf Smith County, TX\"\t48117\t\"Oldham County, TX\"\t48359\n\"Deaf Smith County, TX\"\t48117\t\"Parmer County, TX\"\t48369\n\"Deaf Smith County, TX\"\t48117\t\"Potter County, TX\"\t48375\n\"Deaf Smith County, TX\"\t48117\t\"Randall County, TX\"\t48381\n\"Delta County, TX\"\t48119\t\"Delta County, TX\"\t48119\n\"Delta County, TX\"\t48119\t\"Fannin County, TX\"\t48147\n\"Delta County, TX\"\t48119\t\"Franklin County, TX\"\t48159\n\"Delta County, TX\"\t48119\t\"Hopkins County, TX\"\t48223\n\"Delta County, TX\"\t48119\t\"Hunt County, TX\"\t48231\n\"Delta County, TX\"\t48119\t\"Lamar County, TX\"\t48277\n\"Delta County, TX\"\t48119\t\"Red River County, TX\"\t48387\n\"Denton County, TX\"\t48121\t\"Collin County, TX\"\t48085\n\"Denton County, TX\"\t48121\t\"Cooke County, TX\"\t48097\n\"Denton County, TX\"\t48121\t\"Dallas County, TX\"\t48113\n\"Denton County, TX\"\t48121\t\"Denton County, TX\"\t48121\n\"Denton County, TX\"\t48121\t\"Grayson County, TX\"\t48181\n\"Denton County, TX\"\t48121\t\"Tarrant County, TX\"\t48439\n\"Denton County, TX\"\t48121\t\"Wise County, TX\"\t48497\n\"DeWitt County, TX\"\t48123\t\"DeWitt County, TX\"\t48123\n\"DeWitt County, TX\"\t48123\t\"Goliad County, TX\"\t48175\n\"DeWitt County, TX\"\t48123\t\"Gonzales County, TX\"\t48177\n\"DeWitt County, TX\"\t48123\t\"Karnes County, TX\"\t48255\n\"DeWitt County, TX\"\t48123\t\"Lavaca County, TX\"\t48285\n\"DeWitt County, TX\"\t48123\t\"Victoria County, TX\"\t48469\n\"Dickens County, TX\"\t48125\t\"Cottle County, TX\"\t48101\n\"Dickens County, TX\"\t48125\t\"Crosby County, TX\"\t48107\n\"Dickens County, TX\"\t48125\t\"Dickens County, TX\"\t48125\n\"Dickens County, TX\"\t48125\t\"Floyd County, TX\"\t48153\n\"Dickens County, TX\"\t48125\t\"Garza County, TX\"\t48169\n\"Dickens County, TX\"\t48125\t\"Kent County, TX\"\t48263\n\"Dickens County, TX\"\t48125\t\"King County, TX\"\t48269\n\"Dickens County, TX\"\t48125\t\"Motley County, TX\"\t48345\n\"Dickens County, TX\"\t48125\t\"Stonewall County, TX\"\t48433\n\"Dimmit County, TX\"\t48127\t\"Dimmit County, TX\"\t48127\n\"Dimmit County, TX\"\t48127\t\"Frio County, TX\"\t48163\n\"Dimmit County, TX\"\t48127\t\"La Salle County, TX\"\t48283\n\"Dimmit County, TX\"\t48127\t\"Maverick County, TX\"\t48323\n\"Dimmit County, TX\"\t48127\t\"Webb County, TX\"\t48479\n\"Dimmit County, TX\"\t48127\t\"Zavala County, TX\"\t48507\n\"Donley County, TX\"\t48129\t\"Armstrong County, TX\"\t48011\n\"Donley County, TX\"\t48129\t\"Briscoe County, TX\"\t48045\n\"Donley County, TX\"\t48129\t\"Carson County, TX\"\t48065\n\"Donley County, TX\"\t48129\t\"Collingsworth County, TX\"\t48087\n\"Donley County, TX\"\t48129\t\"Donley County, TX\"\t48129\n\"Donley County, TX\"\t48129\t\"Gray County, TX\"\t48179\n\"Donley County, TX\"\t48129\t\"Hall County, TX\"\t48191\n\"Donley County, TX\"\t48129\t\"Wheeler County, TX\"\t48483\n\"Duval County, TX\"\t48131\t\"Brooks County, TX\"\t48047\n\"Duval County, TX\"\t48131\t\"Duval County, TX\"\t48131\n\"Duval County, TX\"\t48131\t\"Jim Hogg County, TX\"\t48247\n\"Duval County, TX\"\t48131\t\"Jim Wells County, TX\"\t48249\n\"Duval County, TX\"\t48131\t\"La Salle County, TX\"\t48283\n\"Duval County, TX\"\t48131\t\"Live Oak County, TX\"\t48297\n\"Duval County, TX\"\t48131\t\"McMullen County, TX\"\t48311\n\"Duval County, TX\"\t48131\t\"Webb County, TX\"\t48479\n\"Eastland County, TX\"\t48133\t\"Brown County, TX\"\t48049\n\"Eastland County, TX\"\t48133\t\"Callahan County, TX\"\t48059\n\"Eastland County, TX\"\t48133\t\"Comanche County, TX\"\t48093\n\"Eastland County, TX\"\t48133\t\"Eastland County, TX\"\t48133\n\"Eastland County, TX\"\t48133\t\"Erath County, TX\"\t48143\n\"Eastland County, TX\"\t48133\t\"Palo Pinto County, TX\"\t48363\n\"Eastland County, TX\"\t48133\t\"Shackelford County, TX\"\t48417\n\"Eastland County, TX\"\t48133\t\"Stephens County, TX\"\t48429\n\"Ector County, TX\"\t48135\t\"Andrews County, TX\"\t48003\n\"Ector County, TX\"\t48135\t\"Crane County, TX\"\t48103\n\"Ector County, TX\"\t48135\t\"Ector County, TX\"\t48135\n\"Ector County, TX\"\t48135\t\"Midland County, TX\"\t48329\n\"Ector County, TX\"\t48135\t\"Upton County, TX\"\t48461\n\"Ector County, TX\"\t48135\t\"Ward County, TX\"\t48475\n\"Ector County, TX\"\t48135\t\"Winkler County, TX\"\t48495\n\"Edwards County, TX\"\t48137\t\"Edwards County, TX\"\t48137\n\"Edwards County, TX\"\t48137\t\"Kerr County, TX\"\t48265\n\"Edwards County, TX\"\t48137\t\"Kimble County, TX\"\t48267\n\"Edwards County, TX\"\t48137\t\"Kinney County, TX\"\t48271\n\"Edwards County, TX\"\t48137\t\"Real County, TX\"\t48385\n\"Edwards County, TX\"\t48137\t\"Sutton County, TX\"\t48435\n\"Edwards County, TX\"\t48137\t\"Uvalde County, TX\"\t48463\n\"Edwards County, TX\"\t48137\t\"Val Verde County, TX\"\t48465\n\"Ellis County, TX\"\t48139\t\"Dallas County, TX\"\t48113\n\"Ellis County, TX\"\t48139\t\"Ellis County, TX\"\t48139\n\"Ellis County, TX\"\t48139\t\"Henderson County, TX\"\t48213\n\"Ellis County, TX\"\t48139\t\"Hill County, TX\"\t48217\n\"Ellis County, TX\"\t48139\t\"Johnson County, TX\"\t48251\n\"Ellis County, TX\"\t48139\t\"Kaufman County, TX\"\t48257\n\"Ellis County, TX\"\t48139\t\"Navarro County, TX\"\t48349\n\"Ellis County, TX\"\t48139\t\"Tarrant County, TX\"\t48439\n\"El Paso County, TX\"\t48141\t\"Do?a Ana County, NM\"\t35013\n\"El Paso County, TX\"\t48141\t\"Otero County, NM\"\t35035\n\"El Paso County, TX\"\t48141\t\"El Paso County, TX\"\t48141\n\"El Paso County, TX\"\t48141\t\"Hudspeth County, TX\"\t48229\n\"Erath County, TX\"\t48143\t\"Bosque County, TX\"\t48035\n\"Erath County, TX\"\t48143\t\"Comanche County, TX\"\t48093\n\"Erath County, TX\"\t48143\t\"Eastland County, TX\"\t48133\n\"Erath County, TX\"\t48143\t\"Erath County, TX\"\t48143\n\"Erath County, TX\"\t48143\t\"Hamilton County, TX\"\t48193\n\"Erath County, TX\"\t48143\t\"Hood County, TX\"\t48221\n\"Erath County, TX\"\t48143\t\"Palo Pinto County, TX\"\t48363\n\"Erath County, TX\"\t48143\t\"Somervell County, TX\"\t48425\n\"Falls County, TX\"\t48145\t\"Bell County, TX\"\t48027\n\"Falls County, TX\"\t48145\t\"Falls County, TX\"\t48145\n\"Falls County, TX\"\t48145\t\"Limestone County, TX\"\t48293\n\"Falls County, TX\"\t48145\t\"McLennan County, TX\"\t48309\n\"Falls County, TX\"\t48145\t\"Milam County, TX\"\t48331\n\"Falls County, TX\"\t48145\t\"Robertson County, TX\"\t48395\n\"Fannin County, TX\"\t48147\t\"Bryan County, OK\"\t40013\n\"Fannin County, TX\"\t48147\t\"Collin County, TX\"\t48085\n\"Fannin County, TX\"\t48147\t\"Delta County, TX\"\t48119\n\"Fannin County, TX\"\t48147\t\"Fannin County, TX\"\t48147\n\"Fannin County, TX\"\t48147\t\"Grayson County, TX\"\t48181\n\"Fannin County, TX\"\t48147\t\"Hunt County, TX\"\t48231\n\"Fannin County, TX\"\t48147\t\"Lamar County, TX\"\t48277\n\"Fayette County, TX\"\t48149\t\"Austin County, TX\"\t48015\n\"Fayette County, TX\"\t48149\t\"Bastrop County, TX\"\t48021\n\"Fayette County, TX\"\t48149\t\"Caldwell County, TX\"\t48055\n\"Fayette County, TX\"\t48149\t\"Colorado County, TX\"\t48089\n\"Fayette County, TX\"\t48149\t\"Fayette County, TX\"\t48149\n\"Fayette County, TX\"\t48149\t\"Gonzales County, TX\"\t48177\n\"Fayette County, TX\"\t48149\t\"Lavaca County, TX\"\t48285\n\"Fayette County, TX\"\t48149\t\"Lee County, TX\"\t48287\n\"Fayette County, TX\"\t48149\t\"Washington County, TX\"\t48477\n\"Fisher County, TX\"\t48151\t\"Fisher County, TX\"\t48151\n\"Fisher County, TX\"\t48151\t\"Jones County, TX\"\t48253\n\"Fisher County, TX\"\t48151\t\"Kent County, TX\"\t48263\n\"Fisher County, TX\"\t48151\t\"Mitchell County, TX\"\t48335\n\"Fisher County, TX\"\t48151\t\"Nolan County, TX\"\t48353\n\"Fisher County, TX\"\t48151\t\"Scurry County, TX\"\t48415\n\"Fisher County, TX\"\t48151\t\"Stonewall County, TX\"\t48433\n\"Fisher County, TX\"\t48151\t\"Taylor County, TX\"\t48441\n\"Floyd County, TX\"\t48153\t\"Briscoe County, TX\"\t48045\n\"Floyd County, TX\"\t48153\t\"Crosby County, TX\"\t48107\n\"Floyd County, TX\"\t48153\t\"Dickens County, TX\"\t48125\n\"Floyd County, TX\"\t48153\t\"Floyd County, TX\"\t48153\n\"Floyd County, TX\"\t48153\t\"Hale County, TX\"\t48189\n\"Floyd County, TX\"\t48153\t\"Lubbock County, TX\"\t48303\n\"Floyd County, TX\"\t48153\t\"Motley County, TX\"\t48345\n\"Floyd County, TX\"\t48153\t\"Swisher County, TX\"\t48437\n\"Foard County, TX\"\t48155\t\"Baylor County, TX\"\t48023\n\"Foard County, TX\"\t48155\t\"Cottle County, TX\"\t48101\n\"Foard County, TX\"\t48155\t\"Foard County, TX\"\t48155\n\"Foard County, TX\"\t48155\t\"Hardeman County, TX\"\t48197\n\"Foard County, TX\"\t48155\t\"King County, TX\"\t48269\n\"Foard County, TX\"\t48155\t\"Knox County, TX\"\t48275\n\"Foard County, TX\"\t48155\t\"Wilbarger County, TX\"\t48487\n\"Fort Bend County, TX\"\t48157\t\"Austin County, TX\"\t48015\n\"Fort Bend County, TX\"\t48157\t\"Brazoria County, TX\"\t48039\n\"Fort Bend County, TX\"\t48157\t\"Fort Bend County, TX\"\t48157\n\"Fort Bend County, TX\"\t48157\t\"Harris County, TX\"\t48201\n\"Fort Bend County, TX\"\t48157\t\"Waller County, TX\"\t48473\n\"Fort Bend County, TX\"\t48157\t\"Wharton County, TX\"\t48481\n\"Franklin County, TX\"\t48159\t\"Camp County, TX\"\t48063\n\"Franklin County, TX\"\t48159\t\"Delta County, TX\"\t48119\n\"Franklin County, TX\"\t48159\t\"Franklin County, TX\"\t48159\n\"Franklin County, TX\"\t48159\t\"Hopkins County, TX\"\t48223\n\"Franklin County, TX\"\t48159\t\"Red River County, TX\"\t48387\n\"Franklin County, TX\"\t48159\t\"Titus County, TX\"\t48449\n\"Franklin County, TX\"\t48159\t\"Wood County, TX\"\t48499\n\"Freestone County, TX\"\t48161\t\"Anderson County, TX\"\t48001\n\"Freestone County, TX\"\t48161\t\"Freestone County, TX\"\t48161\n\"Freestone County, TX\"\t48161\t\"Henderson County, TX\"\t48213\n\"Freestone County, TX\"\t48161\t\"Leon County, TX\"\t48289\n\"Freestone County, TX\"\t48161\t\"Limestone County, TX\"\t48293\n\"Freestone County, TX\"\t48161\t\"Navarro County, TX\"\t48349\n\"Frio County, TX\"\t48163\t\"Atascosa County, TX\"\t48013\n\"Frio County, TX\"\t48163\t\"Dimmit County, TX\"\t48127\n\"Frio County, TX\"\t48163\t\"Frio County, TX\"\t48163\n\"Frio County, TX\"\t48163\t\"La Salle County, TX\"\t48283\n\"Frio County, TX\"\t48163\t\"Medina County, TX\"\t48325\n\"Frio County, TX\"\t48163\t\"Uvalde County, TX\"\t48463\n\"Frio County, TX\"\t48163\t\"Zavala County, TX\"\t48507\n\"Gaines County, TX\"\t48165\t\"Lea County, NM\"\t35025\n\"Gaines County, TX\"\t48165\t\"Andrews County, TX\"\t48003\n\"Gaines County, TX\"\t48165\t\"Dawson County, TX\"\t48115\n\"Gaines County, TX\"\t48165\t\"Gaines County, TX\"\t48165\n\"Gaines County, TX\"\t48165\t\"Martin County, TX\"\t48317\n\"Gaines County, TX\"\t48165\t\"Terry County, TX\"\t48445\n\"Gaines County, TX\"\t48165\t\"Yoakum County, TX\"\t48501\n\"Galveston County, TX\"\t48167\t\"Brazoria County, TX\"\t48039\n\"Galveston County, TX\"\t48167\t\"Chambers County, TX\"\t48071\n\"Galveston County, TX\"\t48167\t\"Galveston County, TX\"\t48167\n\"Galveston County, TX\"\t48167\t\"Harris County, TX\"\t48201\n\"Garza County, TX\"\t48169\t\"Borden County, TX\"\t48033\n\"Garza County, TX\"\t48169\t\"Crosby County, TX\"\t48107\n\"Garza County, TX\"\t48169\t\"Dickens County, TX\"\t48125\n\"Garza County, TX\"\t48169\t\"Garza County, TX\"\t48169\n\"Garza County, TX\"\t48169\t\"Kent County, TX\"\t48263\n\"Garza County, TX\"\t48169\t\"Lubbock County, TX\"\t48303\n\"Garza County, TX\"\t48169\t\"Lynn County, TX\"\t48305\n\"Garza County, TX\"\t48169\t\"Scurry County, TX\"\t48415\n\"Gillespie County, TX\"\t48171\t\"Blanco County, TX\"\t48031\n\"Gillespie County, TX\"\t48171\t\"Gillespie County, TX\"\t48171\n\"Gillespie County, TX\"\t48171\t\"Kendall County, TX\"\t48259\n\"Gillespie County, TX\"\t48171\t\"Kerr County, TX\"\t48265\n\"Gillespie County, TX\"\t48171\t\"Kimble County, TX\"\t48267\n\"Gillespie County, TX\"\t48171\t\"Llano County, TX\"\t48299\n\"Gillespie County, TX\"\t48171\t\"Mason County, TX\"\t48319\n\"Glasscock County, TX\"\t48173\t\"Glasscock County, TX\"\t48173\n\"Glasscock County, TX\"\t48173\t\"Howard County, TX\"\t48227\n\"Glasscock County, TX\"\t48173\t\"Martin
